vi "newton_eqn.vi"(4 "dt":dbl, 6 "v_Earth_init":dbl, 7 "b1_s0":dbl caption="body1_initial_pos", 10 "b1_m":dbl caption="body1_mass", 11 "F":dbl caption="Force") -> (3 "b1_s1":dbl caption="body1_final_pos")   [LabVIEW 2020]
panel:
  # "Equation of Newtonian Gravity\nF = G*(m1*m2)/r^2\n\nF=m*a\nint(int(F)) = m*s\n    ,where s = position\n                G = 6.674e-11 m^3*kg^-1*s*-2 \nds = v * t\ns = v1*t + (1/2)*a*t^2\ns = v1*t + (1/2)*(F/m)*t^2"
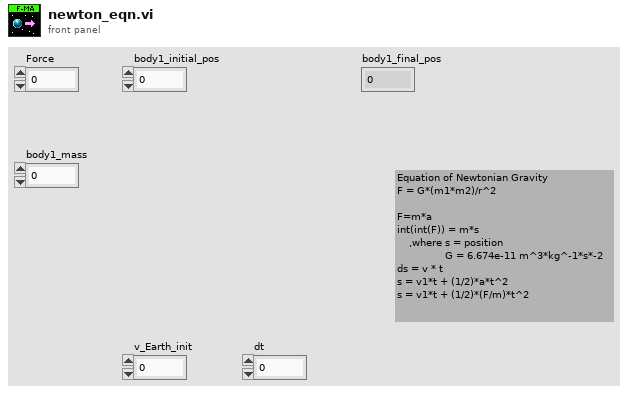
[diagram p1: front panel]
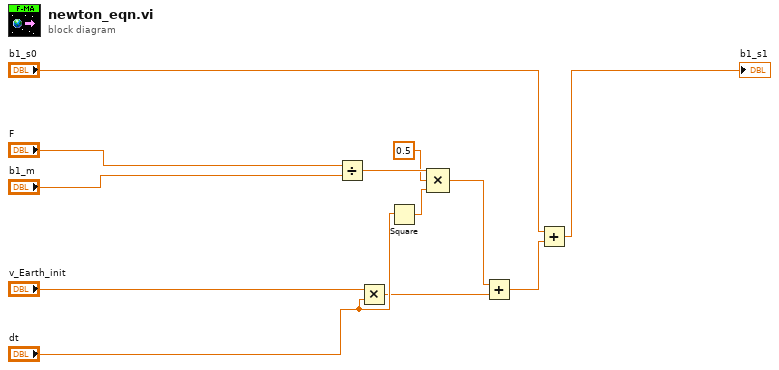
[diagram p0: block diagram]
diagram:
  n1 = Divide(x="F", y="b1_m") -> (x/y=w6:dbl)
  n2 = Multiply(x="v_Earth_init", y="dt") -> (x*y=w2:dbl)
  n3 = Square(x="dt") -> (x^2=w7:dbl)
  n4 = Compound Arithmetic op=MULTIPLY(w6, 0.5 ("Numeric 3"), w7) -> (w8:dbl)
  n5 = Add(x=w8, y=w2) -> (x+y=w9:dbl)
  n6 = Add(x="b1_s0", y=w9) -> (x+y=→"b1_s1":dbl)
